vi "ClsConfigureSetValues.vi"(8 "error in (no error)":errorcluster, 9 "NewVal":i32, 10 "string":string, 11 "Connection Out in":u32) -> (0 "Response":i32, 2 "error out":errorcluster, 3 "Connection Out out":u32)   [LabVIEW 2015]
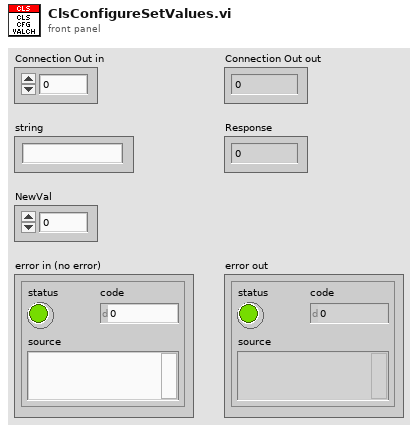
[diagram p1: front panel]
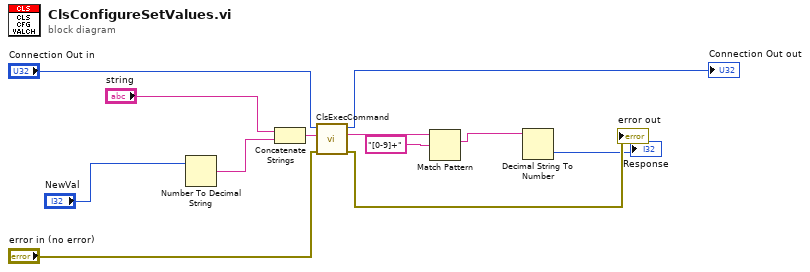
[diagram p0: block diagram]
diagram:
  n1 = Number To Decimal String(number="NewVal") -> (decimal integer string=w3:string)  [unwired: 1 in]
  n2 = Concatenate Strings("string", w3) -> (w2:string)
  n3 = call "ClsExecCommand.vi"("error in (no error)"="error in (no error)", "Command In"=w2, "Connection In"="Connection Out in") -> ("error out"=→"error out":errorcluster, "Command Response"=w8:string, "Connection Out"=→"Connection Out out":u32)  [unwired: 6 in]
  n4 = Match Pattern(string=w8, regular expression="[0-9]+") -> (match substring=w10:string)  [unwired: 1 in, 3 out]
  n5 = Decimal String To Number(string=w10) -> (number=→"Response":i32)  [unwired: 2 in, 1 out]
